vi "DHE_GetControllerStatus.vi"() -> (1 "dhe string":string, 2 "ControllerStatus":T1={"Response"="", "power"=TRUE, "shutter"=FALSE, "artifdata"=FALSE, "idlemode"=FALSE, "reset"=FALSE, "gain"=0, "speed"=0, "resetPCI"=FALSE, "autoshutter"=FALSE, "TempSetPoint"=-110, "multipleextensions"=TRUE, "displayImage"=TRUE, "coadding"=FALSE, "images being coadded"=1, "Operation Mode"=enum."normal", "frames to write"={"subs"=FALSE, "reset"=FALSE, "exposed"=FALSE}, "fawler samples"=1, "write auto"=TRUE, "datatype"="", "frames to display"={"subs"=FALSE, "reset"=FALSE, "exposed"=FALSE}, "sur"=1, "autoclear"=FALSE})   [LabVIEW 2016]
uses:
  Common/public/vis/CMN_ContStatus.ctl
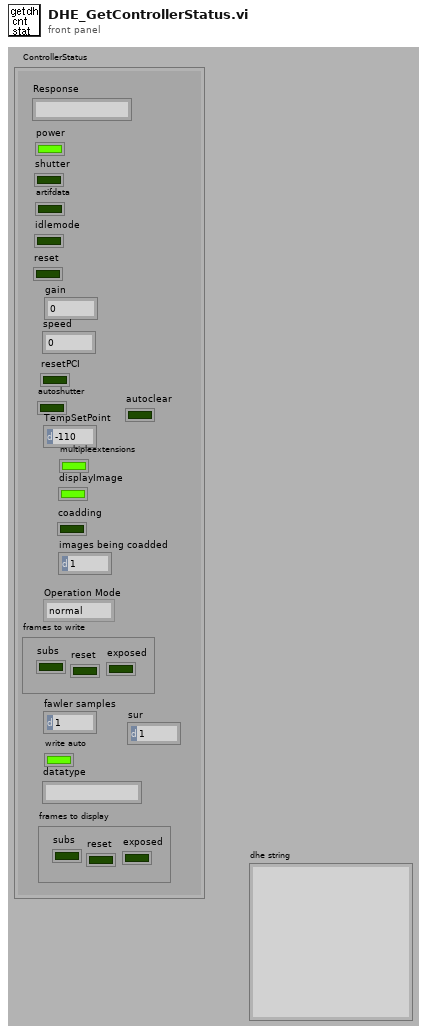
[diagram p1: front panel]
types:
  T1 = typedef "CMN_ContStatus.ctl" = cluster{"Response":string, "power":bool, "shutter":bool, "artifdata":bool, "idlemode":bool, "reset":bool, "gain":u8, "speed":u8, "resetPCI":bool, "autoshutter":bool, "TempSetPoint":i32, "multipleextensions":bool, "displayImage":bool, "coadding":bool, "images being coadded":i32, "Operation Mode":enum16{"normal", "coadd", "fawler"}, "frames to write":cluster{"subs":bool, "reset":bool, "exposed":bool}, "fawler samples":i32, "write auto":bool, "datatype":string, "frames to display":cluster{"subs":bool, "reset":bool, "exposed":bool}, "sur":i32, "autoclear":bool}
  T2 = typedef "DatabaseHand_RefNum.ctl" = refnum<vi>
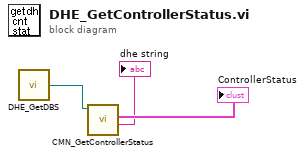
[diagram p0: block diagram]
diagram:
  n1 = call "DHE_GetDBS.vi"() -> ("DHE_DBSRef"=w1:T2)  [unwired: 9 out]
  n2 = call "CMN_GetControllerStatus.vi"("DBS Ref"=w1) -> ("dhe string"=→"dhe string":string, "ControllerStatus"=→"ControllerStatus":T1)  [unwired: 9 out]
